vi "Quick Start - Runs - Add Data.vi"   [LabVIEW 2020]
uses:
  Nominal Client/Nominal Client.lvclass
  19192e5f-c46e-4483-8f4d-33940d6cf31d.vi
  Run/Run.lvclass
  Nominal Client/asset.get[].vi
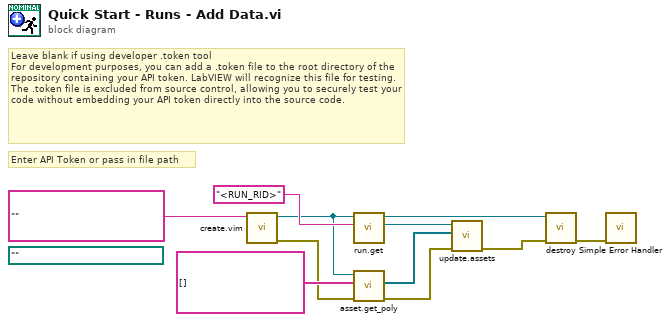
[diagram p0: block diagram]
diagram:
  (unwired) path ""
  # "Leave blank if using developer .token tool\nFor development purposes, you can add a .token file to the root directory of the repository containing your API token. LabVIEW will recognize this file for testing. The .token file is excluded from source control, allowing you to securely test your code without embedding your API token directly into the source code."
  # "Enter API Token or pass in file path"
  n1 = call "create.vim"("API Token (string or path)"="" ("API Token")) -> ("error out"=w4:errorcluster, "Nominal Client"=w3:refnum<class "Nominal Client.lvclass">)  [unwired: 9 in]
  n2 = call "run.get.vi"("Run RID"="<RUN_RID>", "Nominal Client in"=w3) -> ("Run"=w8:refnum<class "Run.lvclass">, "Nominal Client out"=w7:refnum<class "Nominal Client.lvclass">)  [unwired: 7 in, 1 out]
  n3 = call-poly "asset.get_poly.vi"("error in"=w4, "Asset RIDs"=string[] [] ("Run RID"), "Nominal Client in"=w3) -> ("error out"=w2:errorcluster, "Assets"=w6:refnum<class "asset.lvclass">[])  [unwired: 6 in, 1 out]
  n4 = call "update.assets.vi"("error in (no error)"=w2, "Assets"=w6, "Run in"=w8) -> ("error out"=w1:errorcluster)  [unwired: 7 in, 1 out]
  n5 = call "destroy.vi"("error in"=w1, "Nominal Client"=w7) -> ("error out"=w10:errorcluster)  [unwired: 9 in]
  n6 = call <vilib>:"Simple Error Handler.vi"("error in (no error)"=w10) -> ()  [unwired: 4 in, 5 out]
